vi "Configure test.vi"(6 "Assert VI Path":path, 7 "Existing Queue Elements":string, 8 "error in (no error)":errorcluster, 11 "Basic Int Equal in":refnum<class "Int Equal.lvclass">) -> (0 "error out":errorcluster)   [LabVIEW 2018, in "Int Equal.lvclass"]
uses:
  Int Equal.lvclass
  10e99f5f-2e56-4dac-a17a-b0931fedb437.vi
  <vilib>/JDP Science/JSONtext/Find Item.vi
  10e99f5f-2e56-4dac-a17a-b0931fedb437.vi/388171de-d4a8-4a1b-9af2-f294fc6ed619.vi
  10e99f5f-2e56-4dac-a17a-b0931fedb437.vi/42b21c7d-3284-4ffd-93ab-ff1e041f8a7e.vi
  <vilib>/JDP Science/JSONtext/String Subset.vi
  Test Class String IDs.vi
  <vilib>/JDP Science/JSONtext/Parsing/Parse Full Path or Item Name.vi
  <vilib>/JDP Science/JSONtext/Offset/Find Item Locations by Path.vi
  <vilib>/JDP Science/JSONtext/JSON text to Variant.vi
  <vilib>/JDP Science/JSONtext/Variant to JSON Text.vi
  <vilib>/JDP Science/JSONtext/Set Item.vi
  Integer.lvclass
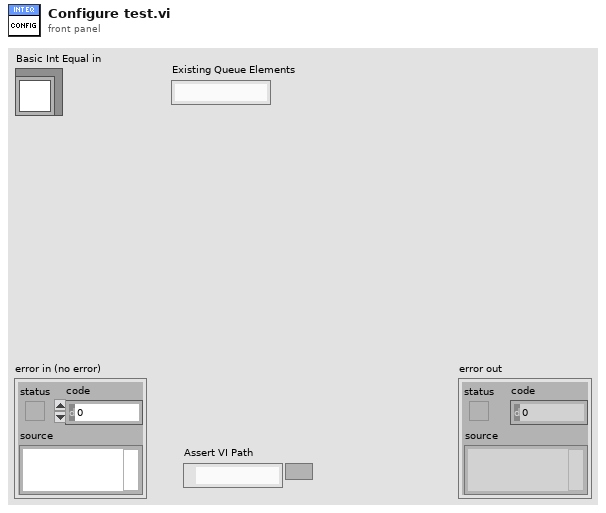
[diagram p1: front panel]
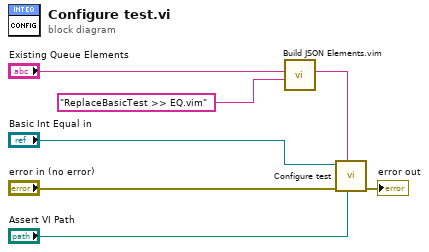
[diagram p0: block diagram]
diagram:
  n1 = call "Build JSON Elements.vim"("Append Element(s)"="ReplaceBasicTest >> EQ.vim", "JSON Elements in ({})"="Existing Queue Elements") -> ("JSON Elements out"=w2:string)  [unwired: 9 in]
  n2 = call-parent "Configure test.vi"("Assert VI Path"="Assert VI Path", "Existing Queue Elements"=w2, "error in (no error)"="error in (no error)", "Basic Integer in"="Basic Int Equal in") -> ("error out"=→"error out":errorcluster)  [unwired: 7 in]
